vi "SelectMenu.vi"(0 "XRef":T16, 1 "Tag":T5, 2 "Point":T15, 3 "Menu Type":T14, 4 "State In":T1) -> (14 "Reply":T13, 15 "Handled?":T9, 16 "Multi Object Popup Options":T12, 17 "Fatal Error Out":T11, 18 "State Out":T1)   [LabVIEW 2021, in "myRIO DO N Samples Open.xnode"]
uses:
  <vilib>/myRIO/Instrument Drivers/Onboard IO/DO Block/vis/myRIO DO N Samples Open.xnode
  <vilib>/XNodeSupport/XNodeXNodeRef.ctl
  <vilib>/XNodeSupport/XNodeString.ctl
  <vilib>/XNodeSupport/XNodePoint.ctl
  <vilib>/XNodeSupport/XNodeInt.ctl
  <vilib>/XNodeSupport/XNodeMenuType.ctl
  <vilib>/myRIO/Instrument Drivers/Onboard IO/DO Block/vis/State.ctl
  <vilib>/myRIO/Common/Instrument Driver Framework/Utilities/typedefs/myRIOXPeripheral.ctl
  <vilib>/XNodeSupport/XNodeTerm4Array.ctl
  <vilib>/XNodeSupport/XNodeTerm4.ctl
  <vilib>/XNodeSupport/XNodeVariant.ctl
  <vilib>/XNodeSupport/XNodeRect32.ctl
  <vilib>/XNodeSupport/XNodeBool.ctl
  <vilib>/XNodeSupport/XNodeTermDirection.ctl
  <vilib>/XNodeSupport/XNodeStringArray.ctl
  <vilib>/XNodeSupport/XNodeMultiObjectPopupOptions.ctl
  <vilib>/XNodeSupport/XNodeErrorCluster.ctl
  <vilib>/XNodeSupport/NI_XNodeSupport.lvlib
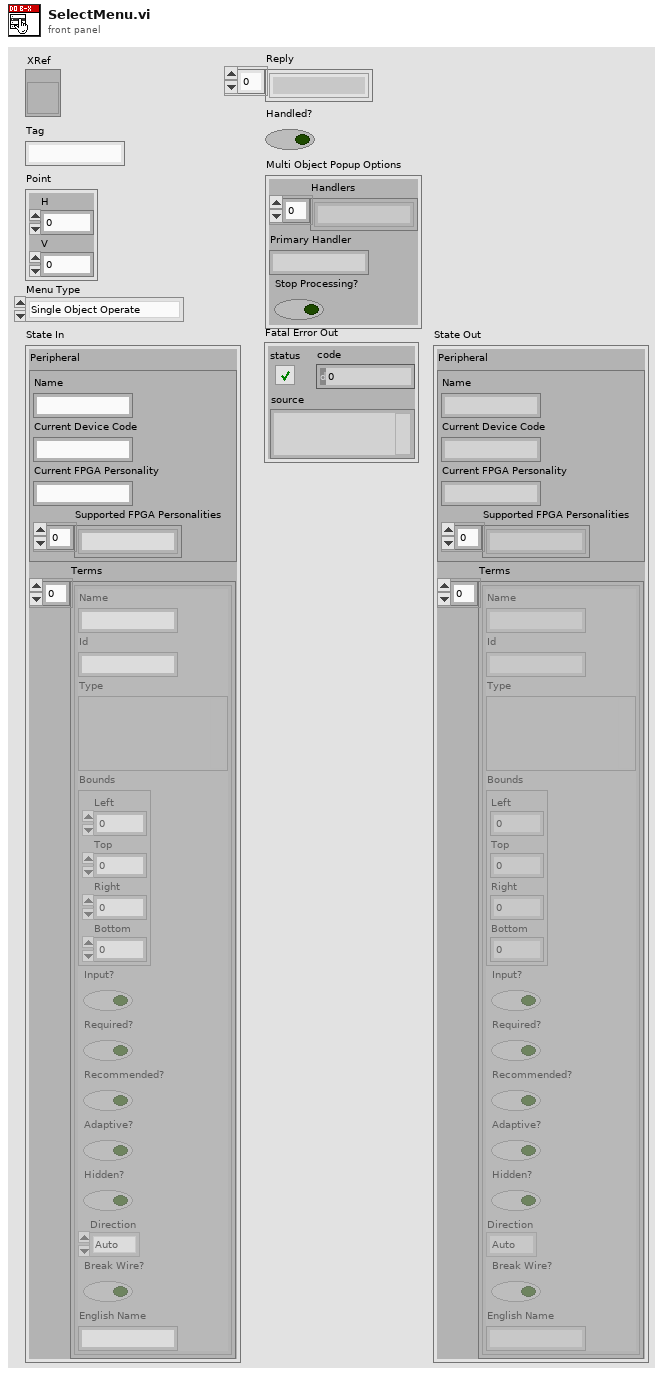
[diagram p1: front panel]
types:
  T1 = typedef "myRIO DO N Samples Open.xnode/State.ctl" = cluster{"Peripheral":T2, "Terms":T3}
  T2 = typedef "myRIOXPeripheral.ctl" = cluster{"Name":string, "Current Device Code":string, "Current FPGA Personality":string, "Supported FPGA Personalities":string[]}
  T3 = typedef "NI_XNodeSupport.lvlib/XNodeTerm4Array.ctl" = T4[]
  T4 = typedef "NI_XNodeSupport.lvlib/XNodeTerm4.ctl" = cluster{"Name":T5, "Id":T5, "Type":T6, "Bounds":T7, "Input?":T9, "Required?":T9, "Recommended?":T9, "Adaptive?":T9, "Hidden?":T9, "Direction":T10, "Break Wire?":T9, "English Name":T5}
  T5 = typedef "NI_XNodeSupport.lvlib/XNodeString.ctl" = string
  T6 = typedef "NI_XNodeSupport.lvlib/XNodeVariant.ctl" = variant
  T7 = typedef "NI_XNodeSupport.lvlib/XNodeRect32.ctl" = cluster{"Left":T8, "Top":T8, "Right":T8, "Bottom":T8}
  T8 = typedef "NI_XNodeSupport.lvlib/XNodeInt.ctl" = i32
  T9 = typedef "NI_XNodeSupport.lvlib/XNodeBool.ctl" = bool
  T10 = typedef "NI_XNodeSupport.lvlib/XNodeTermDirection.ctl" = enum32{"Auto", "Up", "Down", "Left", "Right", "Center"}
  T11 = typedef "NI_XNodeSupport.lvlib/XNodeErrorCluster.ctl" = errorcluster
  T12 = typedef "NI_XNodeSupport.lvlib/XNodeMultiObjectPopupOptions.ctl" = cluster{"Handlers":T13, "Primary Handler":T5, "Stop Processing?":T9}
  T13 = typedef "NI_XNodeSupport.lvlib/XNodeStringArray.ctl" = T5[]
  T14 = typedef "NI_XNodeSupport.lvlib/XNodeMenuType.ctl" = enum32{"Single Object Operate", "Single Object Popup", "Multi Object Popup Master", "Multi Object Popup Other"}
  T15 = typedef "NI_XNodeSupport.lvlib/XNodePoint.ctl" = cluster{"H":T8, "V":T8}
  T16 = typedef "NI_XNodeSupport.lvlib/XNodeXNodeRef.ctl" = refnum<vi>
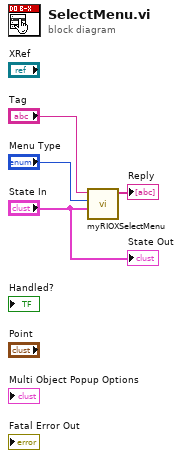
[diagram p0: block diagram]
diagram:
  n1 = call <vilib>:"myRIOXSelectMenu.vi"("State In"="State In", "Menu Type"="Menu Type", "Tag"="Tag") -> ("Reply"=→"Reply":T13)  [unwired: 8 in]
  "State Out" <- "State In"
